vi "Shooter_Globals.vi"() -> ()   [LabVIEW 2020]
uses:
  Subsystems/Cowl/Cowl_States.ctl
  Subsystems/Cowl/Cowl_Cluster.ctl
  Utility VIs/Basic_Motor_Modes.ctl
  Subsystems/Turret/Turret_States.ctl
  Subsystems/Turret/Turret_Cluster.ctl
  Subsystems/Turret/Turret_Motor_Mode.ctl
  Subsystems/Flywheel/Flywheel_States.ctl
  Subsystems/Flywheel/Flywheel_Cluster.ctl
  Shooter_Control_States.ctl
  Determiner_Begin_Cluster.ctl
panel:
  in  "Shooter_Determiner_Set_Ref":string="Shooter_Determiner_Set_Ref"
  in  "Shooter_Determiner_Notifier":refnum<notifier>
  in  "Flywheel_Output":dbl
  in  "Motor_Mode 2":T1
  out "Spun_Up":bool
  in  "Flywheel_Execute_Notifier":refnum<notifier>
  in  "Flywheel_Execute_Ref":string="Flywheel_Execute_Ref"
  in  "Flywheel_Left":string="Flywheel_Left"
  in  "Flywheel_Right":string="Flywheel_Right"
  in  "Turret_Spin_Output":dbl
  in  "Motor_Mode":T2
  out "Turret_Locked":bool
  in  "Turret_CANcoder":string="Turret_CANcoder"
  in  "Turret_Spin":string="Turret_Spin"
  in  "Turret_Execute_Notifier":refnum<notifier>
  in  "Turret_Execute_Ref":string="Turret_Execute_Ref"
  out "Cowl_Absolute_Position (Degrees)":dbl
  out "Cowl_Goal":dbl
  in  "Basic_Motor_Mode":T1
  out "Cowl_Output":dbl
  in  "Cowl_Execute_Notifier":refnum<notifier>
  in  "Cowl_Execute_Ref":string="Cowl_Execute_Ref"
  # "Cowl_globals"
  # "Turret_Globals"
  # "Flywheel_Globals"
  # "Limelight"
  # "Pose"
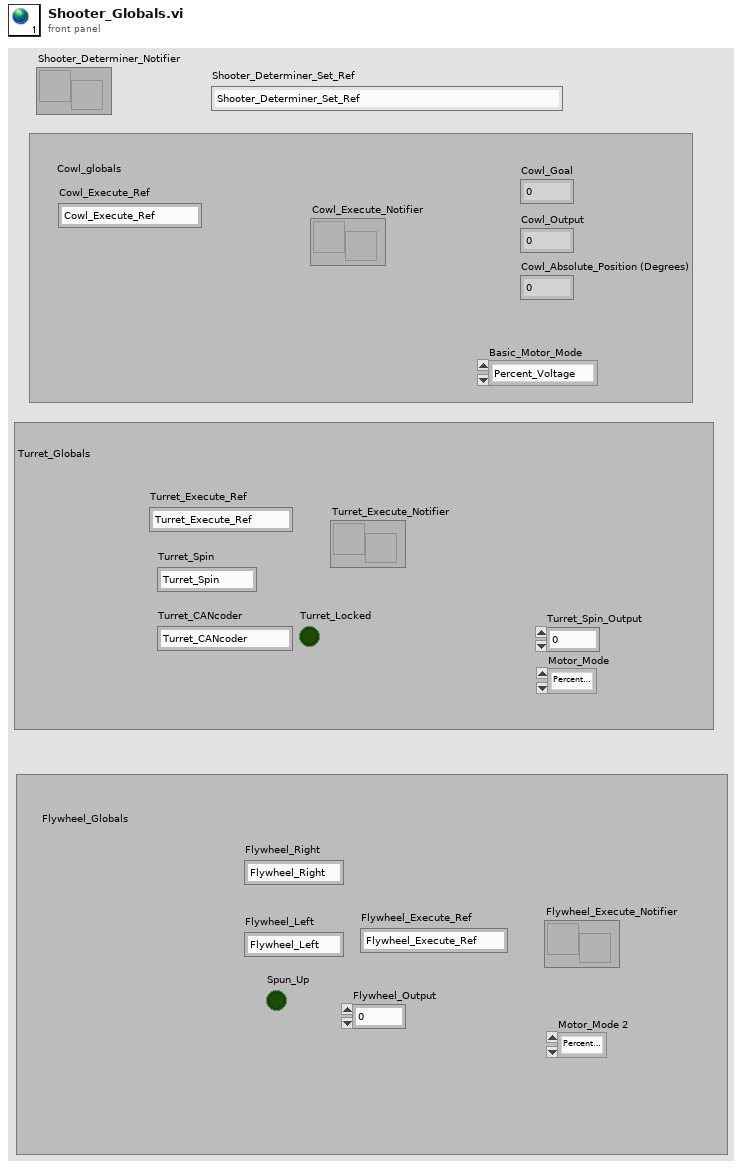
[diagram p1: front panel]
types:
  T1 = typedef "Basic_Motor_Modes.ctl" = enum16{"Percent_Voltage", "Speed_Control", "Position_Control", "Current"}
  T2 = typedef "Turret_Motor_Mode.ctl" = enum16{"Percent_Voltage", "Speed_Control", "Position_Control", "Current"}
diagram:
